vi "SeqMgr.Sequence Load.vi"(8 "error in":errorcluster, 10 "Seq Source Search Folders":path[](array[path]), 11 "File Path":path) -> (0 "error out":errorcluster, 1 "PN":string, 2 "Name":string, 3 "Seq Steps":string[][](array[string]), 4 "Ver":string)   [LabVIEW 2024, in "EQMF.lvlib" / "SeqMgr.lvlib"]
uses:
  SeqMgr.lvlib
  <vilib>/Utility/error.llb/Trim Whitespace One-Sided.vi
  Files/File Utils.lvlib
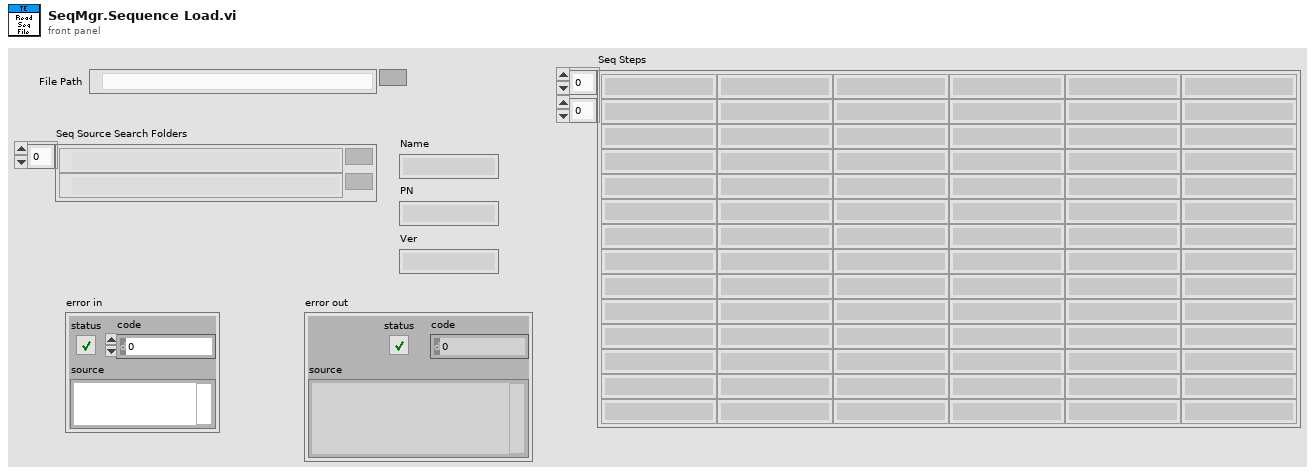
[diagram p1: front panel]
types:
  T1 = cluster{"Steps":string[][], "Name":string, "PN":string, "Ver":string}
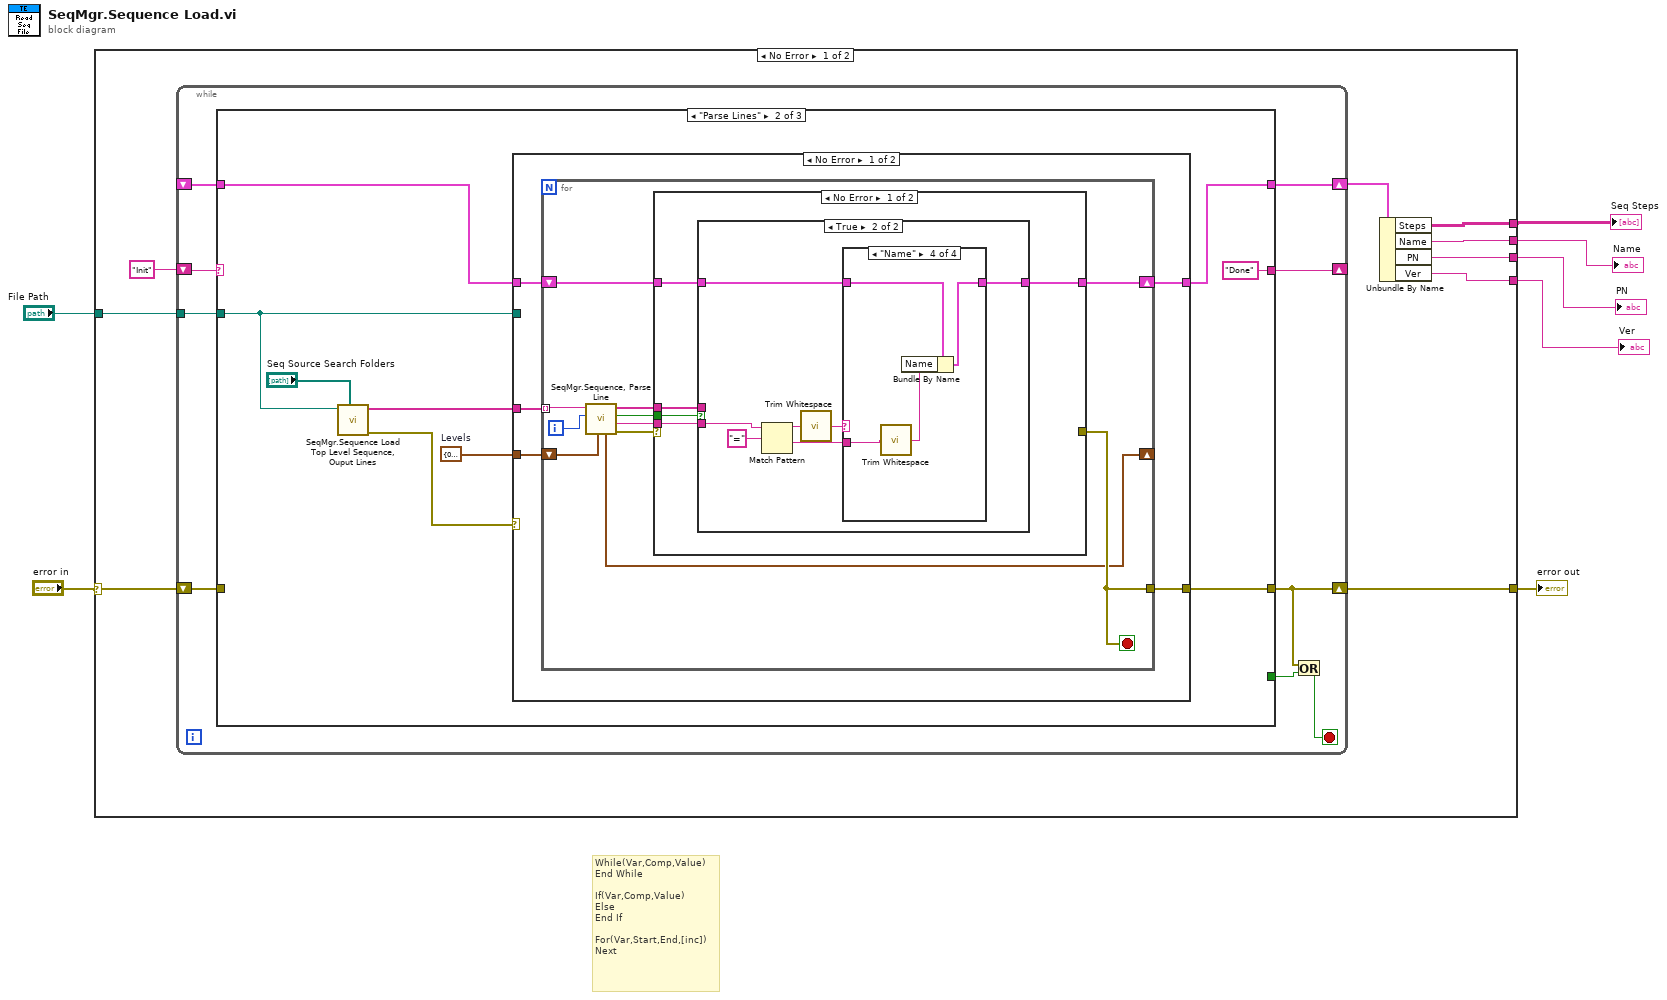
[diagram p0: block diagram]
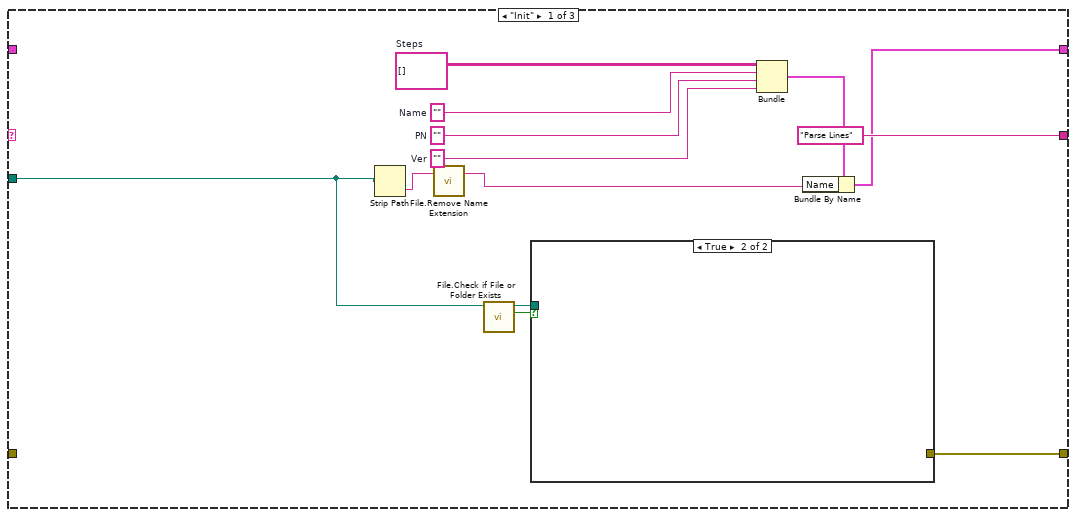
[diagram p2: hidden frame]
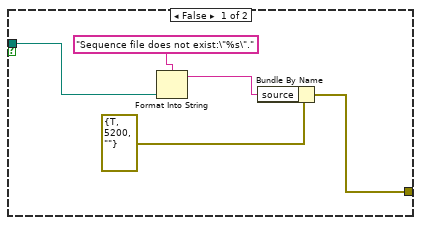
[diagram p3: hidden frame]
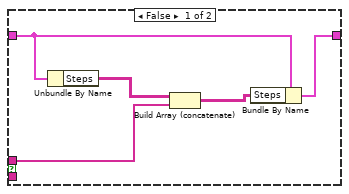
[diagram p4: hidden frame]
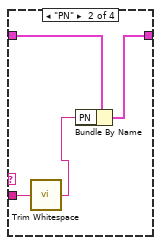
[diagram p6: hidden frame]
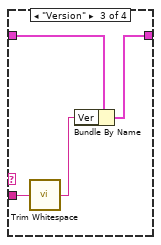
[diagram p7: hidden frame]
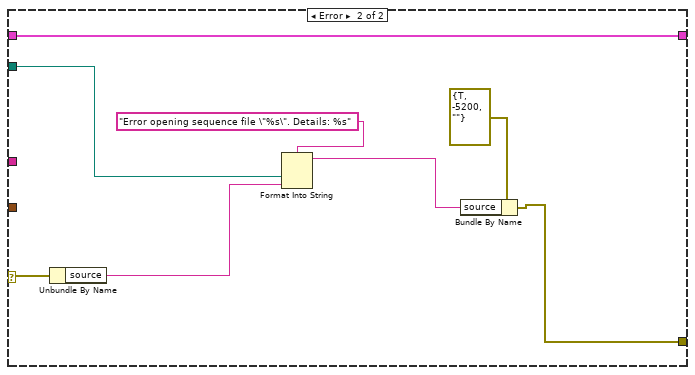
[diagram p9: hidden frame]
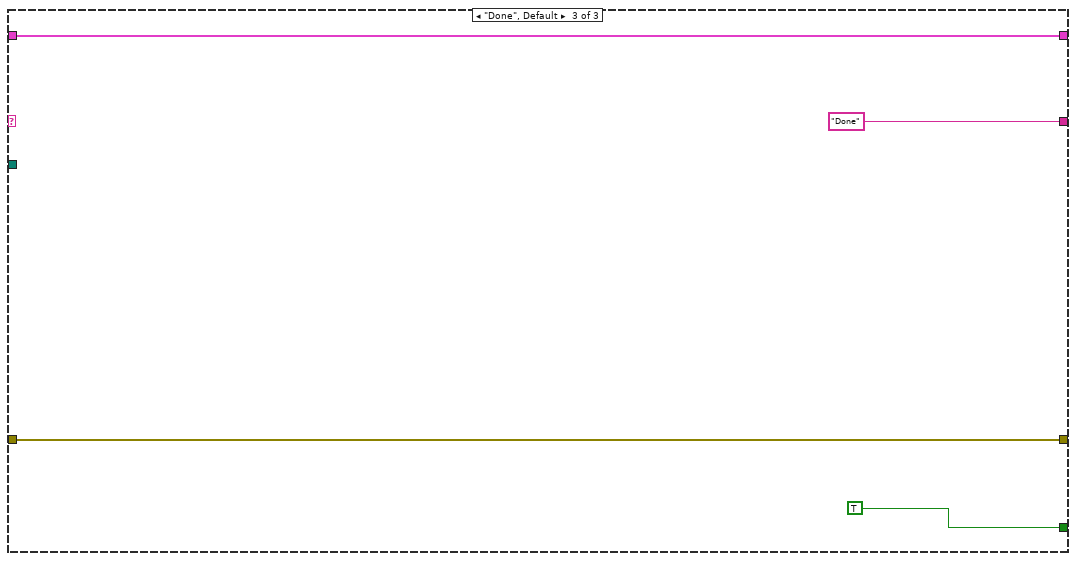
[diagram p10: hidden frame]
diagram:
  # "While(Var,Comp,Value)\nEnd While\n\nIf(Var,Comp,Value)\nElse\nEnd If\n\nFor(Var,Start,End,[inc])\nNext"
  n1 = case shown="No Error" "error in" {
    selector: "error in" -> [w15 w113]
    tunnel: [w14 w113] -> w6
    tunnel: [w12 _] -> w5
    tunnel: [w11 _] -> w4
    tunnel: [w10 _] -> w3
    tunnel: [w9 _] -> w2
    tunnel: "File Path" -> [w8 _]
    frame No Error {
      n2 = while {
        shift-right: [w22] -> w14
        shift-left: w15 -> [w24]
        shift-right: [w18] -> w13
        shift-left: _ -> [w19]
        shift-right: [w20] -> _
        shift-left: "Init" -> [w25]
        tunnel: w8 -> [w17]
        stop <- w21 stop-if-true
        n3 = case shown="\"Parse Lines\"" w25 {
          tunnel: w24 -> [_ _ w111]
          tunnel: [_ _ TRUE] -> w23
          tunnel: [w32 w50 w111] -> w22
          tunnel: ["Parse Lines" "Done" "Done"] -> w20
          tunnel: w19 -> [_ w52 w109]
          tunnel: [w26 w51 w109] -> w18
          tunnel: w17 -> [w30 w45 _]
          frame "Init" {
            w35 = string[][] []  # Steps
            w36 = ""  # Ver
            w37 = ""  # PN
            w38 = ""  # Name
            n4 = Strip Path(path=w30) -> (name=w29:string)  [unwired: 1 out]
            n5 = call "File.Remove Name Extension.vi"("File Name"=w29) -> ("Name Less Ext"=w28:string)  [unwired: 1 in, 1 out]
            n6 = call "File.Check if File or Folder Exists.vi"("Path"=w30) -> ("Exists"=w34:bool, "Dup Path"=w33:path)  [unwired: 6 in, 3 out]
            n7 = case shown="True" w34 {
              tunnel: w33 -> [w42 _]
              tunnel: [w39 _] -> w32
              frame False {
                n8 = Format Into String(format string="Sequence file does not exist:\"%s\".", w42) -> (resulting string=w40:string)  [unwired: 2 in, 1 out]
                n9 = Bundle By Name(cluster=errorcluster {"status"=TRUE, "code"=5200, "source"=""} ("error constant"), "source"=w40) -> (w39:errorcluster)
              }
              frame True {
              }
            }
            n10 = Bundle("Steps"=w35, "Name"=w38, "PN"=w37, "Ver"=w36) -> (w27:T1)  [unwired: 1 in]
            n11 = Bundle By Name(cluster=w27, "Name"=w28) -> (w26:T1)
          }
          frame "Parse Lines" {
            w48 = cluster{"If":i32, "For":i32, "While":i32} {"If"=0, "For"=0, "While"=0}  # Levels
            n12 = call "SeqMgr.Sequence Load Top Level Sequence, Ouput Lines.vi"("Search Folders"="Seq Source Search Folders", "Top Script File"=w45) -> ("Error Out"=w46:errorcluster, "Lines Output"=w47:string[])  [unwired: 8 in]
            n13 = case shown="No Error" w46 {
              selector: w46 -> [_ w105]
              tunnel: w47 -> [w57 _]
              tunnel: w52 -> [w56 w108]
              tunnel: [w54 w108] -> w51
              tunnel: [w55 w106] -> w50
              tunnel: w48 -> [w53 _]
              tunnel: w45 -> [_ w102]
              frame No Error {
                n14 = for {
                  tunnel: w57 -> [w68] mode=indexing
                  tunnel: [w63] -> w55
                  shift-right: [w61] -> w54
                  shift-left: w56 -> [w62]
                  shift-right: [w59] -> _
                  shift-left: w53 -> [w60]
                  i -> [w58]
                  stop <- w63 stop-if-true
                  n15 = call "SeqMgr.Sequence, Parse Line.vi"("Levels"=w60, "LineCnt"=w58, "Line"=w68) -> ("error out"=w67:errorcluster, "Comment"=w64:string, "Is Comment"=w65:bool, "Step"=w66:string[], "Levels Out"=w59:cluster{"If":i32, "For":i32, "While":i32})  [unwired: 4 in]
                  n16 = case shown="No Error" w67 {
                    selector: w67 -> [_ w100]
                    tunnel: w66 -> [w72 _]
                    tunnel: w65 -> [w73 _]
                    tunnel: w64 -> [w71 _]
                    tunnel: [_ w100] -> w63
                    tunnel: w62 -> [w70 w99]
                    tunnel: [w69 w99] -> w61
                    frame No Error {
                      n17 = case shown="True" w73 {
                        tunnel: w72 -> [w78 _]
                        tunnel: w71 -> [_ w84]
                        tunnel: w70 -> [w76 w81]
                        tunnel: [w74 w80] -> w69
                        frame False {
                          n18 = Unbundle By Name(w76) -> ("Steps"=w77:string[][])
                          n19 = Build Array (concatenate)(w77, w78) -> (w75:string[][])
                          n20 = Bundle By Name(cluster=w76, "Steps"=w75) -> (w74:T1)
                        }
                        frame True {
                          n21 = Match Pattern(string=w84, regular expression="=") -> (before substring=w83:string, after substring=w79:string)  [unwired: 1 in, 2 out]
                          n22 = call <vilib>:"Trim Whitespace.vi"("string"=w83) -> ("trimmed string"=w82:string)  [unwired: 1 in]
                          n23 = case shown="\"Name\"" w82 {
                            tunnel: w81 -> [w86 w90 w94 w98]
                            tunnel: [w86 w89 w93 w97] -> w80
                            tunnel: w79 -> [_ w88 w92 w96]
                            frame Default {
                            }
                            frame "PN" {
                              n24 = call <vilib>:"Trim Whitespace.vi"("string"=w88) -> ("trimmed string"=w87:string)  [unwired: 1 in]
                              n25 = Bundle By Name(cluster=w90, "PN"=w87) -> (w89:T1)
                            }
                            frame "Version" {
                              n26 = call <vilib>:"Trim Whitespace.vi"("string"=w92) -> ("trimmed string"=w91:string)  [unwired: 1 in]
                              n27 = Bundle By Name(cluster=w94, "Ver"=w91) -> (w93:T1)
                            }
                            frame "Name" {
                              n28 = call <vilib>:"Trim Whitespace.vi"("string"=w96) -> ("trimmed string"=w95:string)  [unwired: 1 in]
                              n29 = Bundle By Name(cluster=w98, "Name"=w95) -> (w97:T1)
                            }
                          }
                        }
                      }
                    }
                    frame Error {
                    }
                  }
                }
              }
              frame Error {
                n30 = Unbundle By Name(w105) -> ("source"=w101:string)
                n31 = Format Into String(format string="Error opening sequence file \"%s\". Details: %s", w102, w101) -> (resulting string=w103:string)  [unwired: 2 in, 1 out]
                n32 = Bundle By Name(cluster=errorcluster {"status"=TRUE, "code"=-5200, "source"=""} ("error constant"), "source"=w103) -> (w106:errorcluster)
              }
            }
          }
          frame "Done", Default {
          }
        }
        n33 = Or(x=w22, y=w23) -> (x .or. y?=w21:bool)
      }
      n34 = Unbundle By Name(w13) -> ("Steps"=w12:string[][], "Name"=w11:string, "PN"=w10:string, "Ver"=w9:string)
    }
    frame Error {
    }
  }
  "error out" <- w6
  "Seq Steps" <- w5
  "PN" <- w3
  "Ver" <- w2
  "Name" <- w4
